vi "20170502127惠雨3.vi"() -> ()   [LabVIEW 2017]
panel:
  out "XY图":cluster{dbl[], dbl[]}(graph)
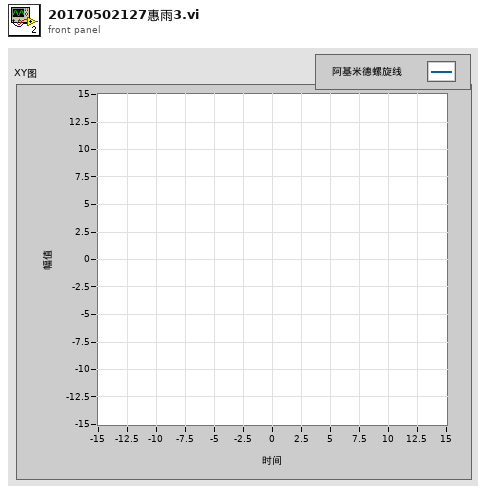
[diagram p1: front panel]
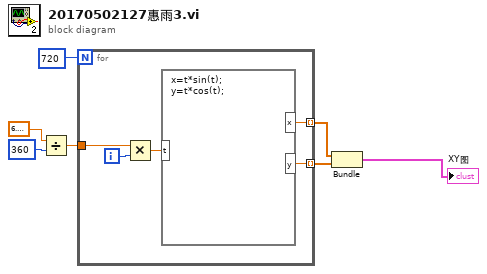
[diagram p0: block diagram]
diagram:
  n1 = Divide(x=6.283185307179586, y=360) -> (x/y=w5:dbl)
  n2 = for {
    N: 720 -> [_]
    tunnel: w5 -> [w12]
    tunnel: [w9] -> w3 mode=indexing
    tunnel: [w8] -> w2 mode=indexing
    i -> [w11]
    n3 = Multiply(x=w12, y=w11) -> (x*y=w10:dbl)
    n4 = formula code="x=t*sin(t);\ny=t*cos(t);"("t"=w10) -> ("x"=w9:dbl, "y"=w8:dbl)
  }
  n5 = Bundle(w3, w2) -> (→"XY图":cluster{dbl[], dbl[]})  [unwired: 1 in]
